vi "basic - Receive Continuous Capture.vi"() -> ()   [LabVIEW 2020]
uses:
  _controls/session_monitor_config.ctl
  _polimorphicInstances/session/Fdx Create Session (RX-Monitor).vi
  _polimorphicInstances/control/Fdx Start (Rx).vi
  _polimorphicInstances/control/Fdx Stop (Rx).vi
  _polimorphicInstances/session/Fdx Close Session (Port).vi
  AIM664LV.lvlib
panel:
  in  "TriggerPosition":u32
  in  "Strobe":u32(ring) items=["FDX_MON_STROBE_DIS", "FDX_MON_STROBE_STOP", "FDX_MON_STROBE_START"]
  in  "CaptureMode":u32(ring) items=["FDX_MON_SINGLE ", "FDX_MON_CONTINUOUS", "FDX_MON_SELECTIVE", "FDX_MON_RECORDING", "FDX_MON_REROS", "FDX_MON_HMU"]
  in  "DefaultCronoMode":u32(ring)=2 items=["FDX_RX_DEFAULT_ENA_CNT", "FDX_RX_DEFAULT_MON_ENA_ALL", "FDX_RX_DEFAULT_MON_ENA_GOOD"]
  in  "Tab Control":enum32{"Package", "Statistics"}(tab)
  out "Synchronized":u32
  out "BytesRead":u32
  out "EntryRead":u32
  out "Data":string[][](table)
  out "Statistics":string[][](table)
  out "GlobalStat Out":T1
  in  "Control":u32(ring) items=["FDX_RX_GS_RES_NO_CNT", "FDX_RX_GS_RES_ALL_CNT", "FDX_RX_GS_RES_ERR_CNT"]
  in  "ReadQualifier (0:full)":u32
  in  "poll time ms":u32=100
  in  "QueueSize MB (1)":u32=1
  out "error out":errorcluster
  out "QueueStatus":T2 {"QueueStatus" items=["FDX_MON_STAT_EMPTY", "FDX_MON_STAT_ FILLED", "FDX_MON_STAT_ FULL", "FDX_MON_STAT_ OVERFLOW", "FDX_MON_STAT_ ERROR"]}
  out "GlobMonSize":u32
  out "PortInitOut":T3={"PortConfig"=0, "PortUsed"=1, "GlobalMemFree"=0, "SharedMemFree"=0} {"PortConfig" items=["FDX_SINGLE", "FDX_REDUNDANT"]}
  out "GlbMonBufferSizeOut":u32
  in  "board":u32
  in  "port":u32=1
  in  "DefaultPayloadMode (Full)":u32(ring) items=["FDX_PAYLOAD_FULL", "FDX_PAYLOAD_IP_EXT", "FDX_PAYLOAD_IP", "FDX_PAYLOAD_MAC"]
  in  "stop":bool
  out "current irig time":T4={"SignOut"=40, "DayOut"=1, "HourOut"=1, "MinOut"=28, "SecondOut"=39, "MilliSecOut"=539, "MicroSecOut"=300, "NanoSecOut"=0, "InfoOut"=0, "Mode"=3}
  out "current time":timestamp
  # "ARINC 664 Receive Continuous Capture"
  # "Overview: It helps to obtain the versions stored in the board.\n\nRequirement: One AIM ARINC-664 board with installed AIM ARINC 664 BSP.\nRestrictions: None.\nInstruction:\n1. Select the Board ID (0 if you have only one board in your system) and the port number. If you want to validate between two ports in one device, you can use tx board and Rx Boardd\n2. Run the VI.\n3. See the result in Current IRIG Time"
  # "Monitor Configuration"
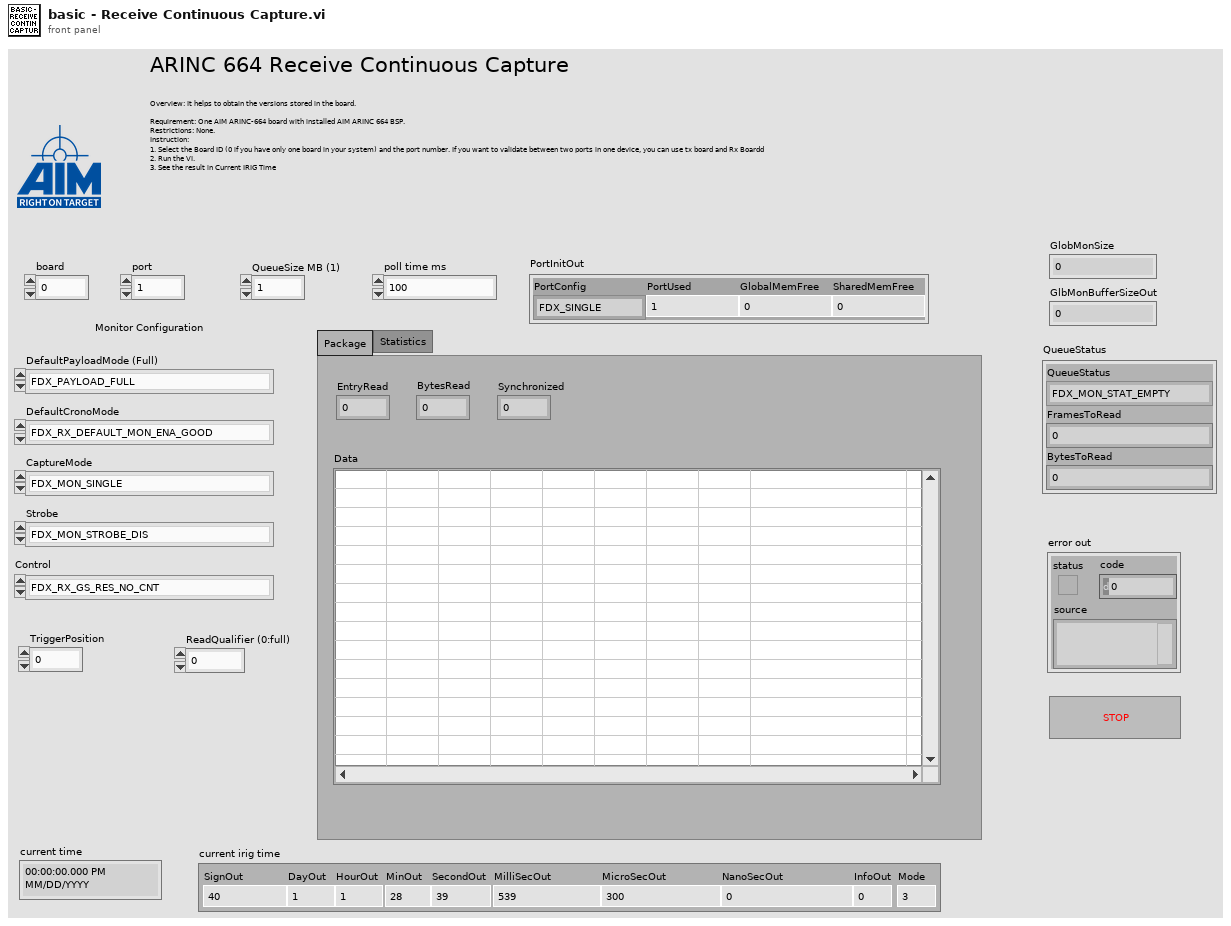
[diagram p1: front panel]
types:
  T1 = cluster{"TotalByteCount":u32[], "FrameGoodCount":u32[], "FrameErrorCount":u32[], "BytesPerSecond":u32[], "FramesPerSecond":u32[], "PhysErrorCount":u32[], "PreamErrorCount":u32[], "UnaligErrorCount":u32[], "CRCErrorCount":u32[], "IFGErrorCount":u32[], "IPErrorCount":u32[], "MACErrorCount":u32[], "NoSfdErrorCount":u32[], "VLLenErrorCount":u32[], "SNIntegrityErrorCount":u32[], "TrafShapingViolationCount":u32[], "MAC1Short":u32[], "MAC64To127Count":u32[], "MAC128To255Count":u32[], "MAC256To511Count":u32[], "MAC512To1023Count":u32[], "MAC1024To1518Count":u32[], "MACLong":u32[]}
  T2 = cluster{"QueueStatus":u32, "FramesToRead":u32, "BytesToRead":u32}
  T3 = cluster{"PortConfig":u32, "PortUsed":u32, "GlobalMemFree":u32, "SharedMemFree":u32}
  T4 = cluster{"SignOut":i32, "DayOut":u32, "HourOut":u32, "MinOut":u32, "SecondOut":u32, "MilliSecOut":u32, "MicroSecOut":u32, "NanoSecOut":u32, "InfoOut":u32, "Mode":u32}
  T5 = typedef "AIM664LV.lvlib/session_monitor_config.ctl" = cluster{"DefaultCronoMode":u32, "GlbMonBufferSizeIn":u32}
  T6 = cluster{"EntryRead":u32, "BytesRead":u32, "Synchronized":u32, "ReadBuffer":u8[]}
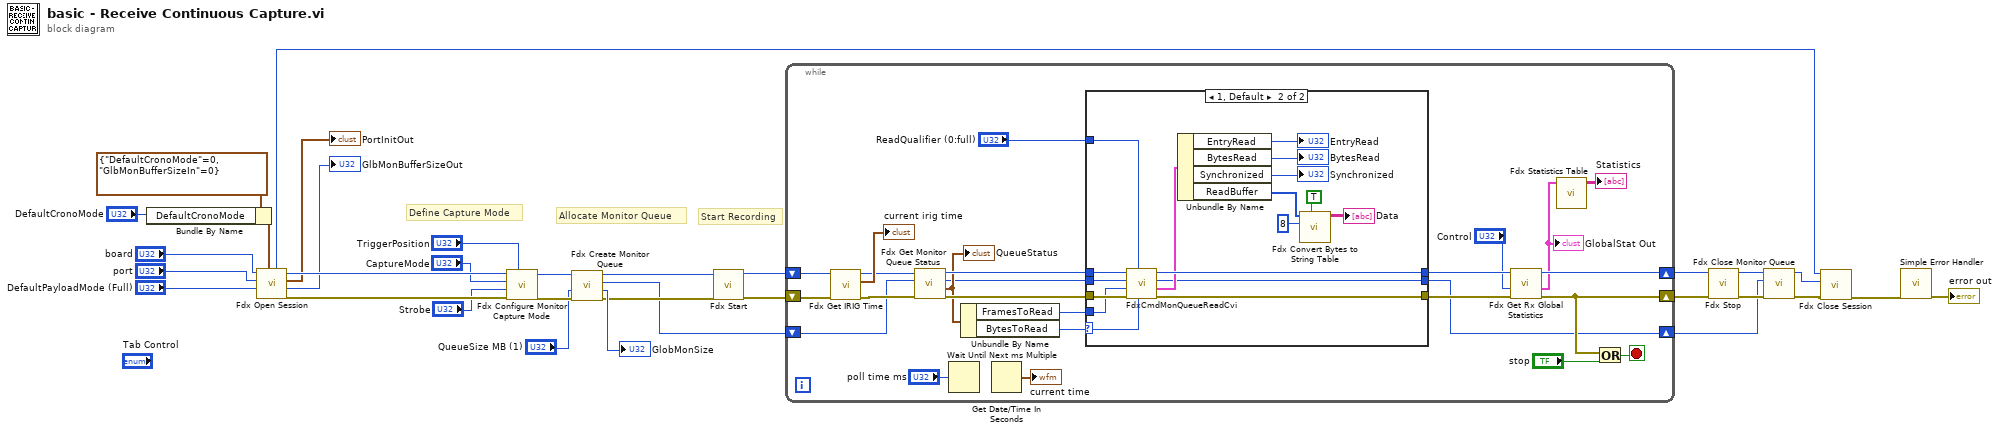
[diagram p0: block diagram]
diagram:
  # "Start Recording"
  # "Allocate Monitor Queue"
  # "Define Capture Mode"
  n1 = Bundle By Name(cluster=T5 {"DefaultCronoMode"=0, "GlbMonBufferSizeIn"=0} ("MonitorConfig"), "DefaultCronoMode"="DefaultCronoMode") -> (w8:T5)
  n2 = call-poly "Fdx Open Session.vi"("MonitorConfig"=w8, "DefaultPayloadMode (Full)"="DefaultPayloadMode (Full)", "port"="port", "board"="board") -> ("error out"=w31:errorcluster, "GlbMonBufferSizeOut"=→"GlbMonBufferSizeOut":u32, "PortInitOut"=→"PortInitOut":T3, "InstrumentHandle_port out"=w32:u32, "InstrumentHandle_board out"=w10:u32)  [unwired: 2 in, 1 out]
  n3 = call "Fdx Configure Monitor Capture Mode.vi"("TriggerPosition"="TriggerPosition", "error in"=w31, "Strobe"="Strobe", "CaptureMode"="CaptureMode", "InstrumentHandle_port in"=w32) -> ("error out"=w29:errorcluster, "InstrumentHandle_port out"=w30:u32)  [unwired: 5 in]
  n4 = call "Fdx Create Monitor Queue.vi"("error in (no error)"=w29, "MaxFileSize MB (1)"="QueueSize MB (1)", "InstrumentHandle_port in"=w30) -> ("error out"=w16:errorcluster, "GlobMonSize"=→"GlobMonSize":u32, "QueueIdOut"=w13:u32, "InstrumentHandle_port out"=w17:u32)  [unwired: 5 in]
  n5 = call-poly "Fdx Start.vi"("error in"=w16, "InstrumentHandle_port in"=w17) -> ("error out"=w22:errorcluster, "InstrumentHandle_port out"=w23:u32)  [unwired: 8 in]
  n6 = while {
    shift-right: [w34] -> w3
    shift-left: w13 -> [w36]
    shift-right: [w42] -> w24
    shift-left: w23 -> [w53]
    shift-right: [w44] -> w18
    shift-left: w22 -> [w52]
    stop <- w57 stop-if-true
    n7 = call "Fdx Get IRIG Time.vi"("error in (no error)"=w52, "InstrumentHandle_board in"=w53) -> ("error out"=w51:errorcluster, "Curent Irig Time"=→"current irig time":T4, "InstrumentHandle_board out"=w47:u32)  [unwired: 7 in]
    n8 = call "Fdx Get Monitor Queue Status.vi"("error in"=w51, "QueueId"=w36, "InstrumentHandle_port"=w47) -> ("error out"=w50:errorcluster, "QueueStatus"=w48:T2, "QueueIdOut"=w35:u32, "InstrumentHandle_port"=w49:u32)  [unwired: 5 in]
    "QueueStatus" <- w48
    n9 = Wait Until Next ms Multiple(millisecond multiple="poll time ms") -> ()  [unwired: 1 out]
    n10 = Unbundle By Name(w48) -> ("FramesToRead"=w33:u32, "BytesToRead"=w40:u32)
    n11 = Get Date/Time In Seconds() -> (seconds since 1Jan1904=→"current time":timestamp)
    n12 = case shown="1, Default" w40 {
      selector: w40 -> [_ w61]
      tunnel: w50 -> [w60 w77]
      tunnel: w49 -> [w59 w76]
      tunnel: w35 -> [w58 w75]
      tunnel: [w59 w74] -> w46
      tunnel: [w60 w73] -> w45
      tunnel: "ReadQualifier (0:full)" -> [_ w72]
      tunnel: w33 -> [_ w71]
      tunnel: [w58 w62] -> w34
      frame 0 {
      }
      frame 1, Default {
        n13 = call "FdxCmdMonQueueReadCvi.vi"("MaxReadBytes"=w61, "ReadQualifier"=w72, "error in"=w77, "EntryCount"=w71, "QueueId"=w75, "InstrumentHandle_port"=w76) -> ("error out"=w73:errorcluster, "QueueReadOut"=w70:T6, "QueueIdOut"=w62:u32, "InstrumentHandle_port"=w74:u32)  [unwired: 2 in]
        n14 = Unbundle By Name(w70) -> ("EntryRead"=→"EntryRead":u32, "BytesRead"=→"BytesRead":u32, "Synchronized"=→"Synchronized":u32, "ReadBuffer"=w67:u8[])
        n15 = call "Fdx Convert Bytes to String Table.vi"("append ASCII column?"=TRUE ("Append ASCII Column?"), "byters per row"=8, "data"=w67) -> ("data table"=→"Data":string[][])  [unwired: 6 in, 2 out]
      }
    }
    n16 = call "Fdx Get Rx Global Statistics.vi"("error in"=w45, "Control"="Control", "InstrumentHandle_port in"=w46) -> ("error out"=w44:errorcluster, "GlobalStat Out"=w39:T1, "InstrumentHandle_port out"=w42:u32)  [unwired: 6 in]
    "GlobalStat Out" <- w39
    n17 = call "Fdx Statistics Table.vi"("GlobalStat Out"=w39) -> ("Table Control"=→"Statistics":string[][])  [unwired: 10 in]
    n18 = Or(x=w44, y="stop") -> (x .or. y?=w57:bool)
  }
  n19 = call-poly "Fdx Stop.vi"("error in"=w18, "InstrumentHandle_port in"=w24) -> ("error out"=w20:errorcluster, "InstrumentHandle_port out"=w12:u32)  [unwired: 8 in]
  n20 = call "Fdx Close Monitor Queue.vi"("error in (no error)"=w20, "QueueId"=w3, "InstrumentHandle_port in"=w12) -> ("error out"=w19:errorcluster, "InstrumentHandle_port out"=w11:u32)  [unwired: 7 in]
  n21 = call-poly "Fdx Close Session.vi"("error in"=w19, "InstrumentHandle_port in"=w11, "InstrumentHandle_board in"=w10) -> ("error out"=w2:errorcluster)  [unwired: 8 in]
  n22 = call <vilib>:"Simple Error Handler.vi"("error in (no error)"=w2) -> ("error out"=→"error out":errorcluster)  [unwired: 4 in, 4 out]
